vi "UTIL Get Directory.vi"(8 "error in (no error)":errorcluster, 11 "Path In":path) -> (0 "error out":errorcluster, 3 "Directory Out":path)   [LabVIEW 2009]
doc: "This utility will strip the path until it gets a directory that contains the parent VI.\n\nAAL 9/09"
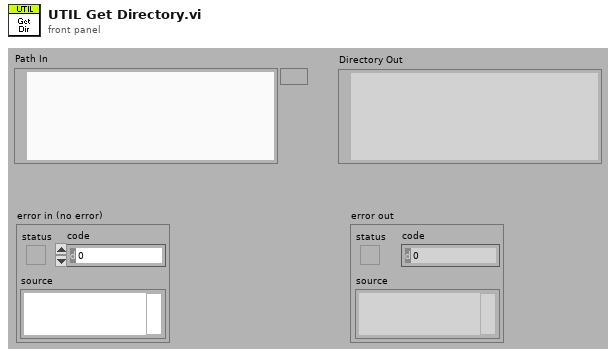
[diagram p1: front panel]
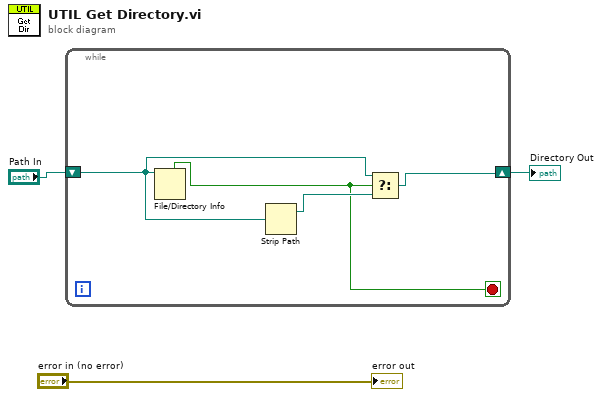
[diagram p0: block diagram]
diagram:
  n1 = while {
    shift-right: [w5] -> w2
    shift-left: "Path In" -> [w7]
    stop <- w4 stop-if-true
    n2 = File/Directory Info(path=w7) -> (directory=w4:bool)  [unwired: 1 in, 6 out]
    n3 = Strip Path(path=w7) -> (stripped path=w6:path)  [unwired: 1 out]
    n4 = Select(t=w7, s=w4, f=w6) -> (s? t:f=w5:path)
  }
  "Directory Out" <- w2
  "error out" <- "error in (no error)"
